vi "Config Measure Delta.vi"(0 "VISA resource name":refnum<visa-resource-name>, 1 "Delta Measure (0: OFF)":u16(ring) items=["OFF", "U1-U2", "I1-I2", "3P3W-3V3A", "Delta-Start", "Start_Delta"], 11 "error in (no error)":errorcluster) -> (4 "VISA resource name out":refnum<visa-resource-name>, 15 "error out":errorcluster)   [LabVIEW 2013, in "Yokogawa PZ4000.lvlib"]
doc: "This VI sends the Delta Measure group command to the PZ4000 series."
uses:
  Yokogawa PZ4000.lvlib
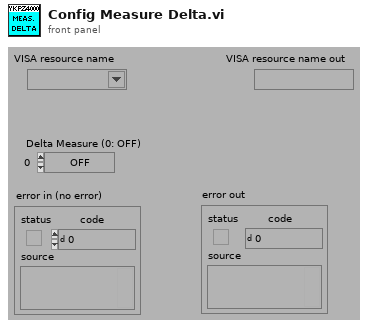
[diagram p1: front panel]
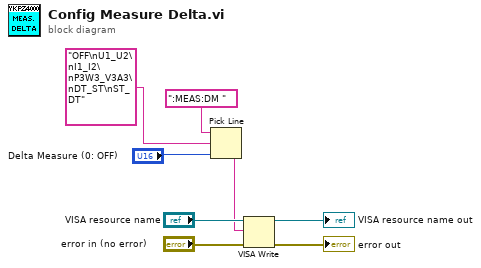
[diagram p0: block diagram]
diagram:
  n1 = Pick Line(string ("")=":MEAS:DM ", multi-line string="OFF\nU1_U2\nI1_I2\nP3W3_V3A3\nDT_ST\nST_DT", line index="Delta Measure (0: OFF)") -> (output string=w1:string)
  n2 = VISA Write(VISA resource name="VISA resource name", write buffer=w1, error in (no error)="error in (no error)") -> (VISA resource name out=→"VISA resource name out":refnum<visa-resource-name>, error out=→"error out":errorcluster)  [unwired: 1 out]
